vi "DockingLine.vi"(1 "X":dbl) -> (0 "Y":dbl)   [LabVIEW 2014]
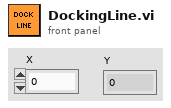
[diagram p1: front panel]
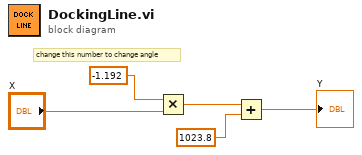
[diagram p0: block diagram]
diagram:
  # "change this number to change angle"
  n1 = Multiply(x=-1.192, y="X") -> (x*y=w3:dbl)
  n2 = Add(x=w3, y=1023.8) -> (x+y=→"Y":dbl)
